vi "LimitSetting.vi"(8 "error in (no error)":errorcluster, 10 "operation":enum16{"Add", "Delete", "Modify"}(ring), 11 "TestSetup in":refnum<class "TestSetup.lvclass">) -> (0 "error out":errorcluster, 3 "TestSetup out":refnum<class "TestSetup.lvclass">)   [LabVIEW 2019, in "TestSetup.lvlib" / "TestSetup.lvclass"]
uses:
  TestSetup.lvclass
  Limit.ctl
  TestSetup.lvclass/TestSetup.ctl
panel:
  in  "OK":bool
  in  "Cancel":bool
  in  "Limit":T1
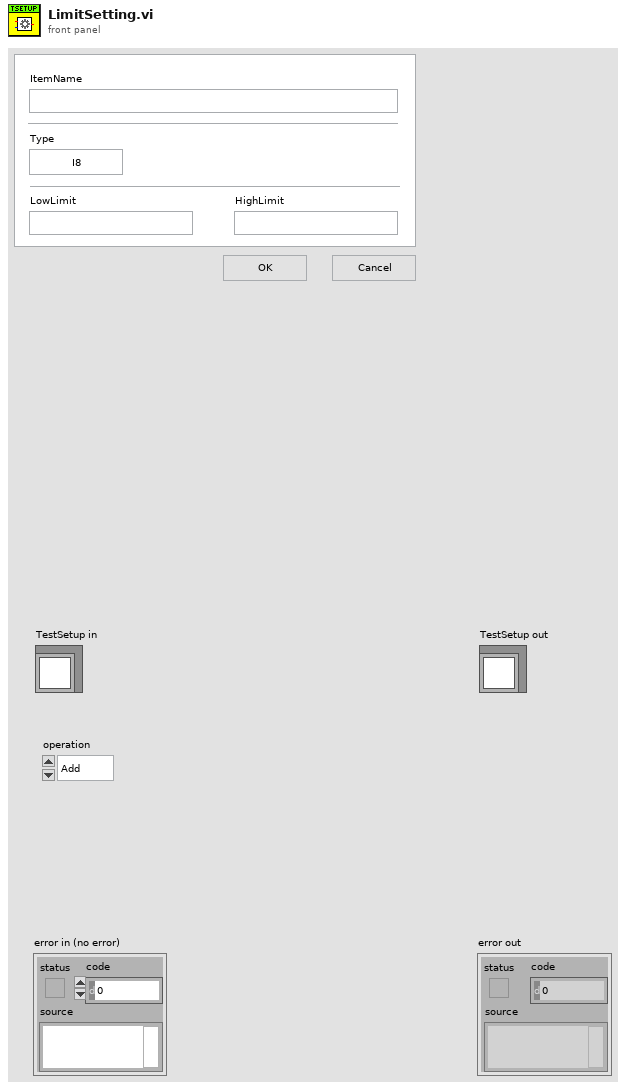
[diagram p1: front panel]
types:
  T1 = typedef "TestSetup.lvlib/TestSetup.lvclass/Limit.ctl" = cluster{"ItemName":string, "Type":enum16{"I8", "I16", "I32", "I64", "U8", "U16", "U32", "U64", "Double Float", "Boolean", "String", "Numeric Array", "String Array"}, "LowLimit":string, "HighLimit":string}
  T2 = enum32{"Invalid", "Standard", "Closed", "Hidden", "Minimized", "Maximized"}
  T3 = enum32{"invalid app kind", "Development System", "Run Time System", "Student Edition", "Embedded LabVIEW", "Evaluation", "Custom"}
  T4 = cluster{"Core":cluster{"Current VI Reference":refnum<vi>, "Close Panel on Exit?":bool}, "Multicolumn Listbox":refnum<vi>, "operation":enum16{"Add", "Delete", "Modify"}, "Limit":refnum<vi>}
  T5 = cluster{"Current VI Reference":refnum<vi>, "Close Panel on Exit?":bool}
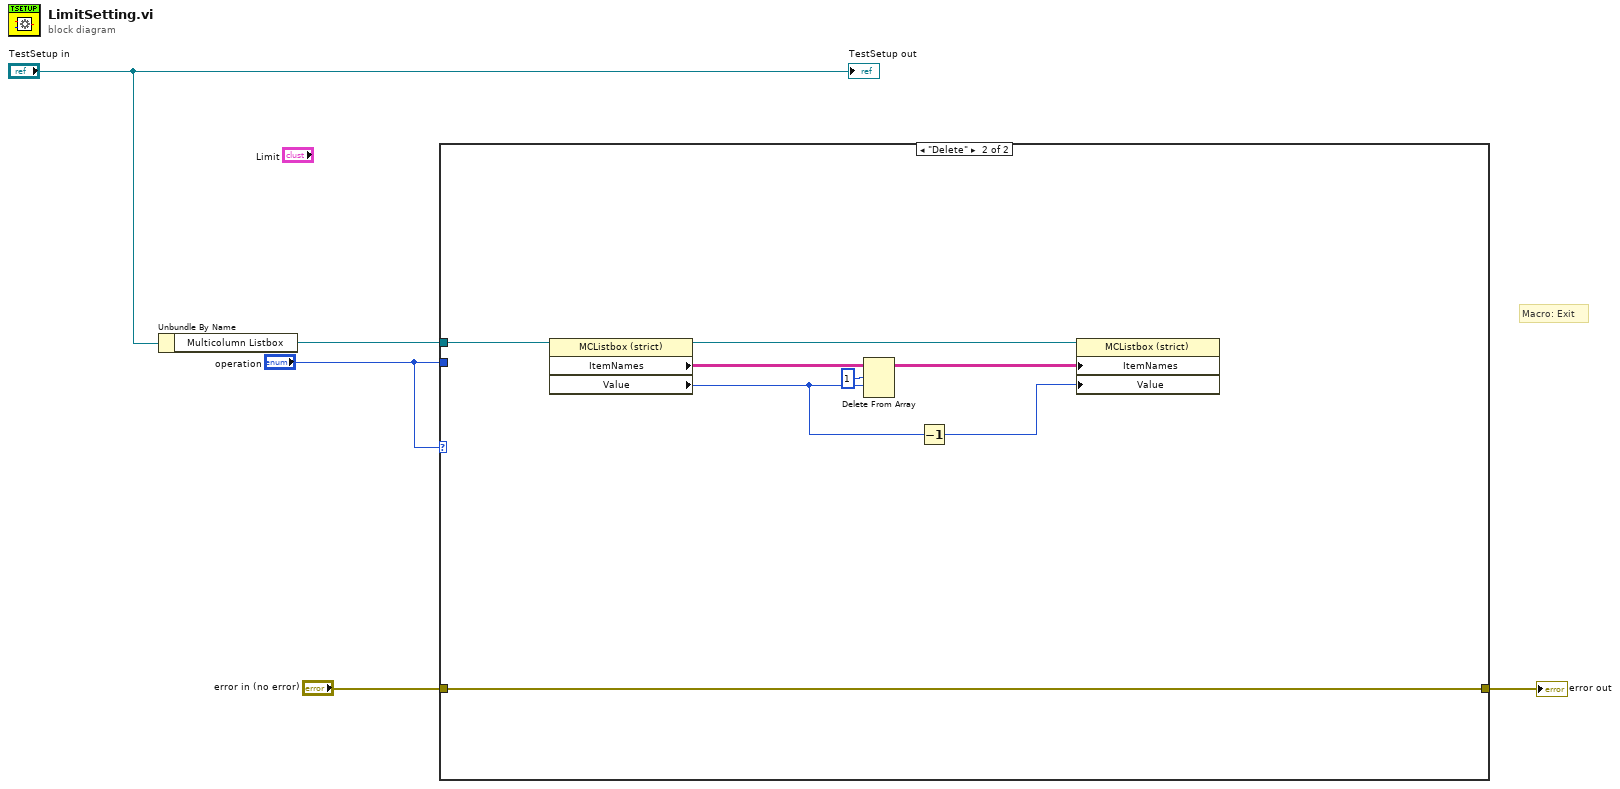
[diagram p0: block diagram]
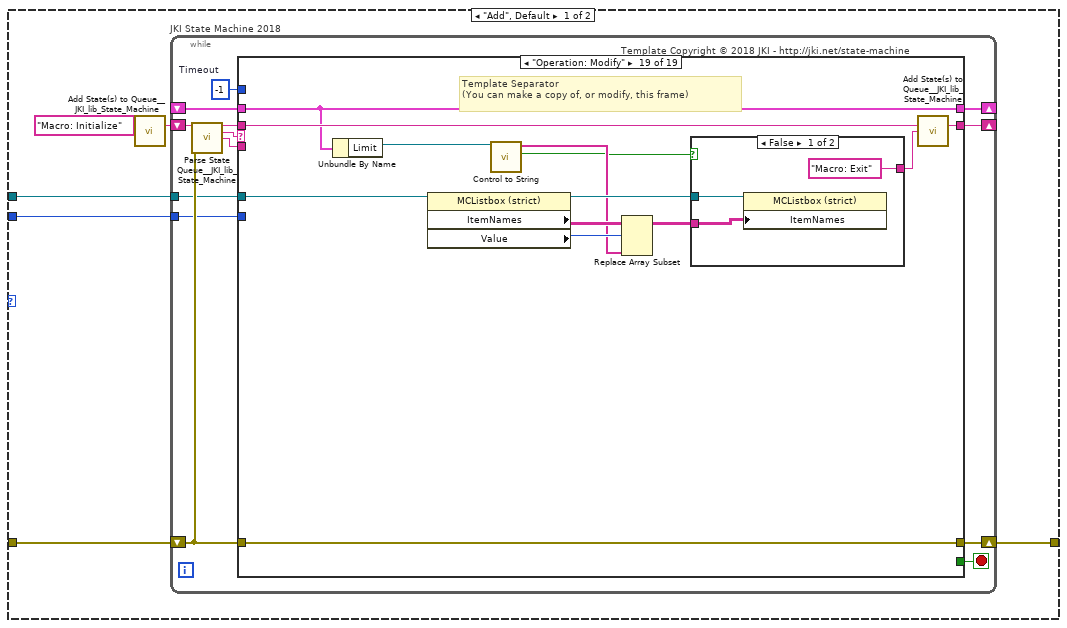
[diagram p2: hidden frame]
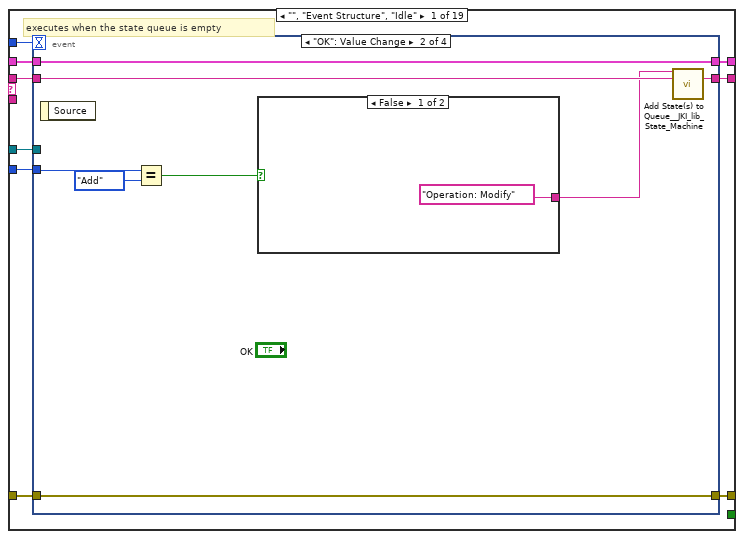
[diagram p3: hidden frame]
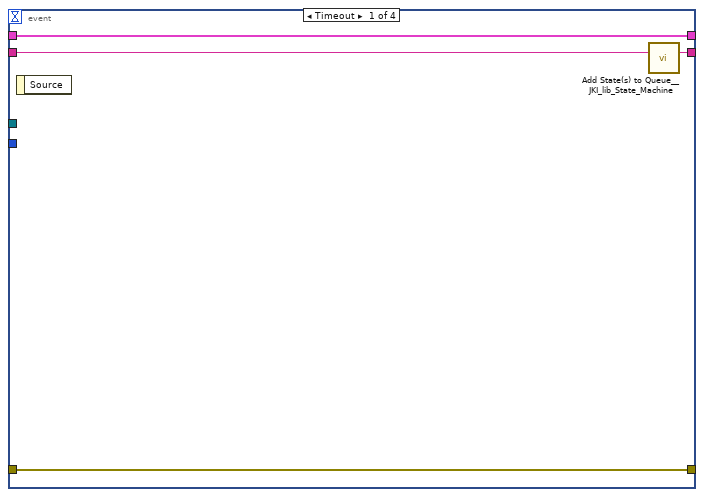
[diagram p4: hidden frame]
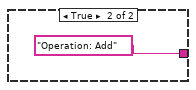
[diagram p5: hidden frame]
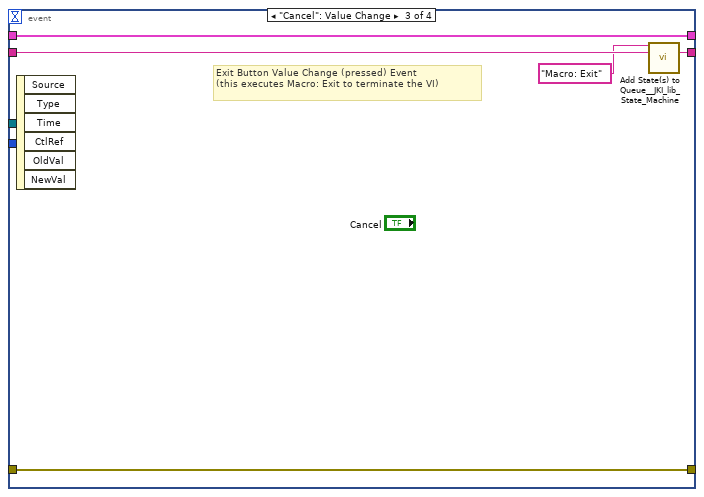
[diagram p6: hidden frame]
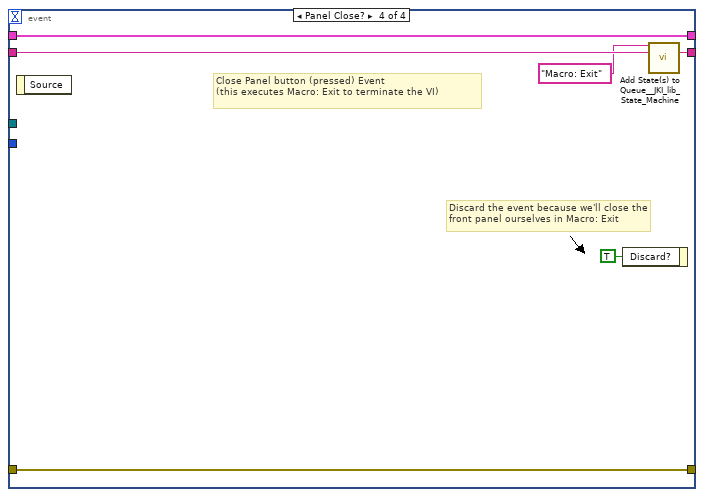
[diagram p7: hidden frame]
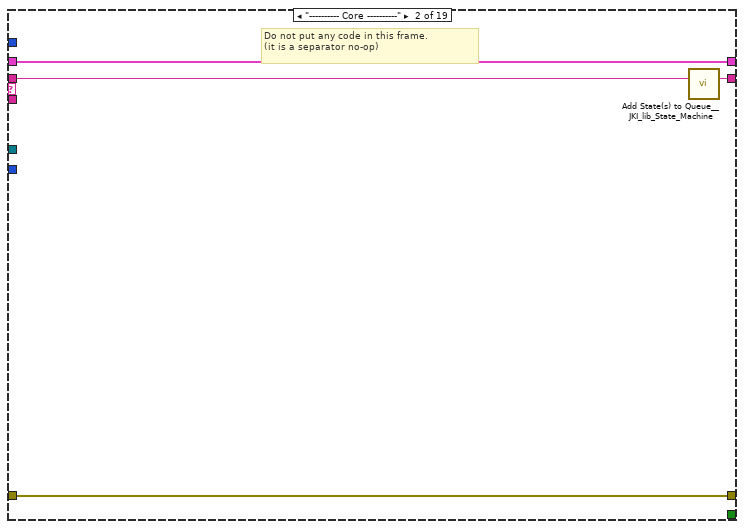
[diagram p8: hidden frame]
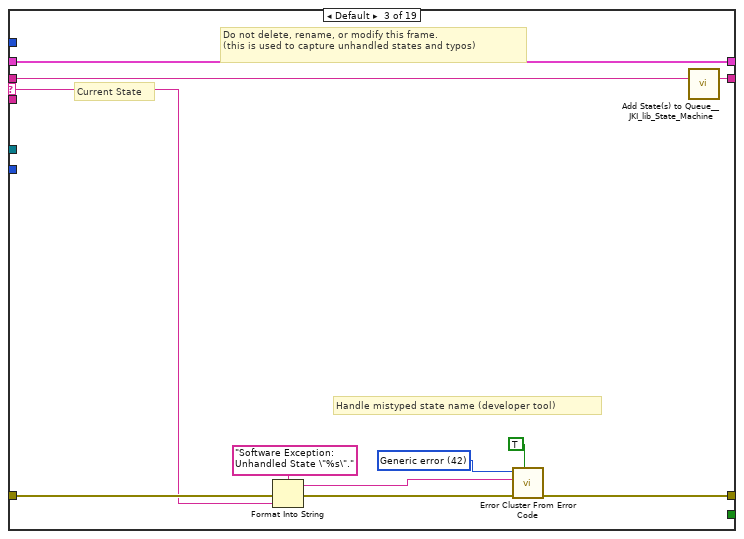
[diagram p9: hidden frame]
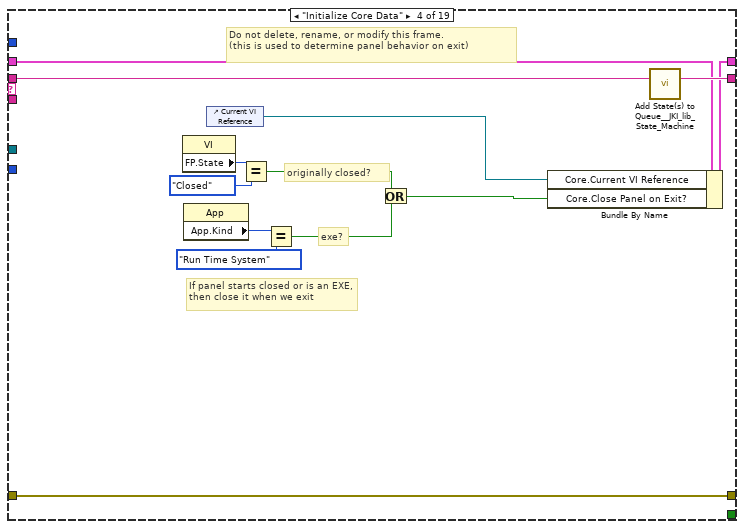
[diagram p10: hidden frame]
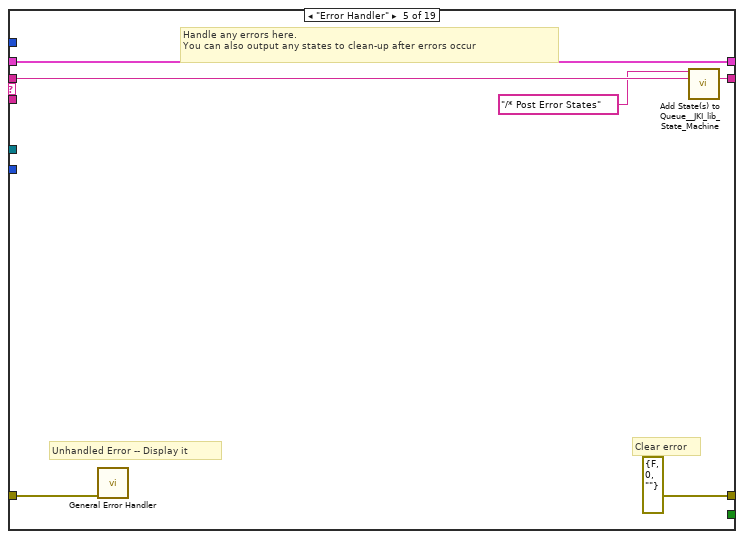
[diagram p11: hidden frame]
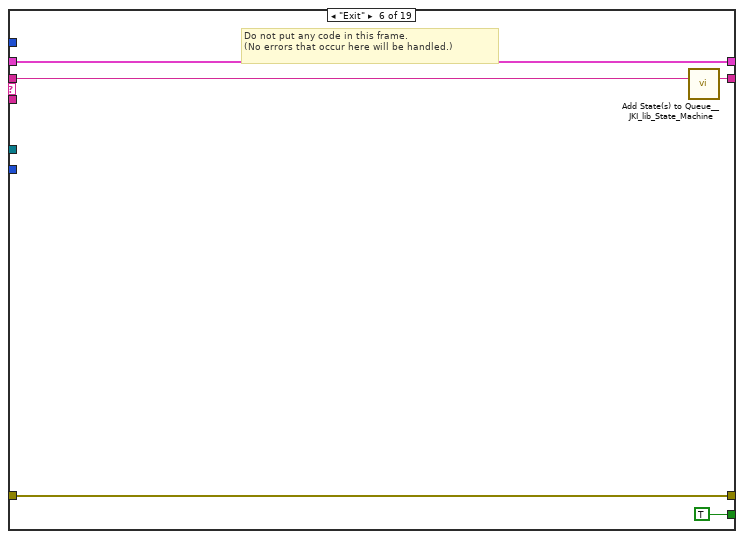
[diagram p12: hidden frame]
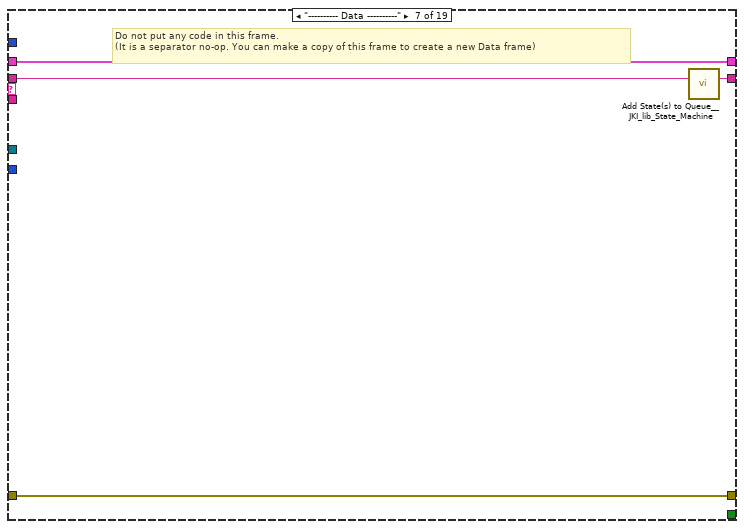
[diagram p13: hidden frame]
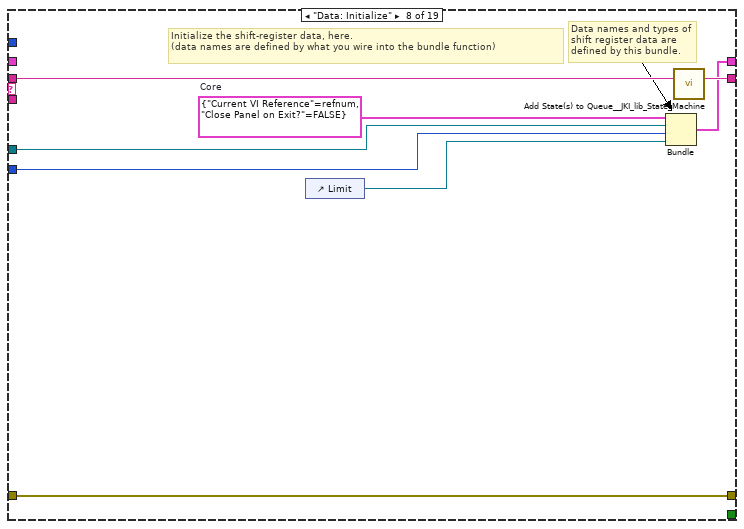
[diagram p14: hidden frame]
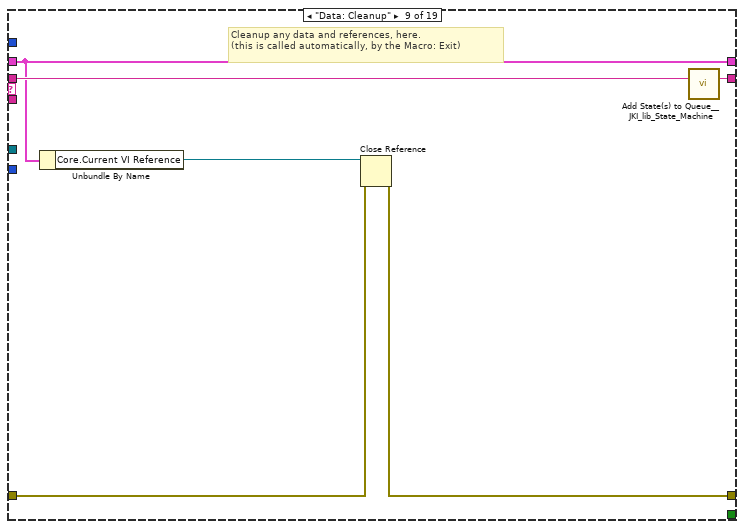
[diagram p15: hidden frame]
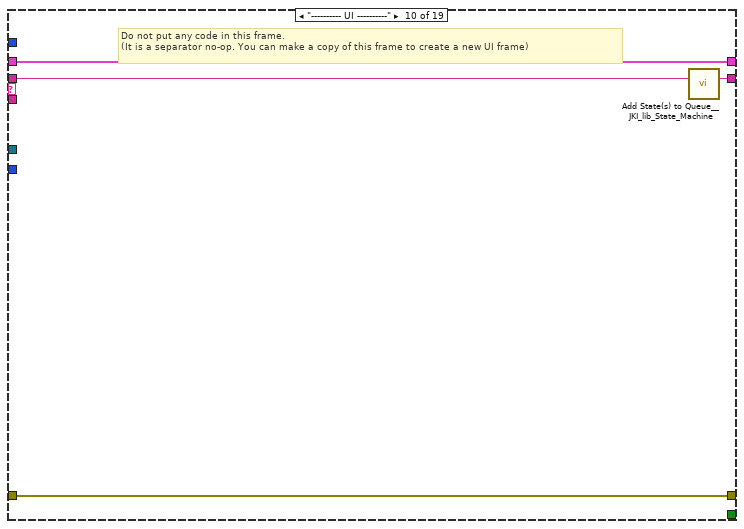
[diagram p16: hidden frame]
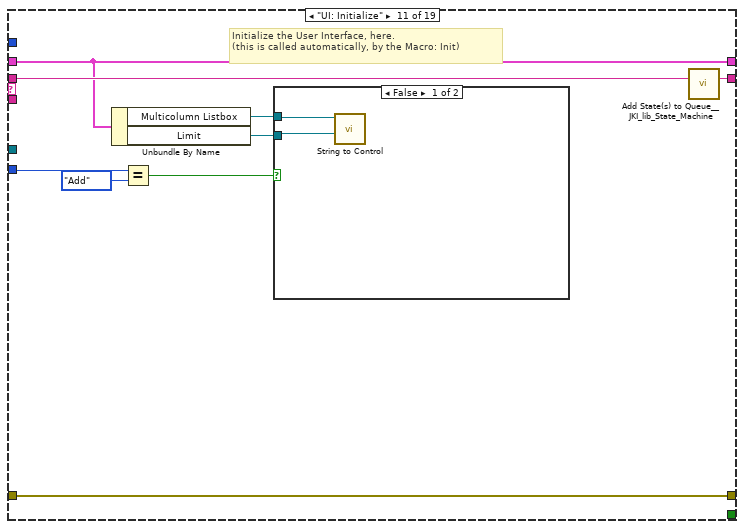
[diagram p17: hidden frame]
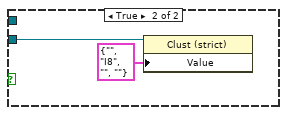
[diagram p18: hidden frame]
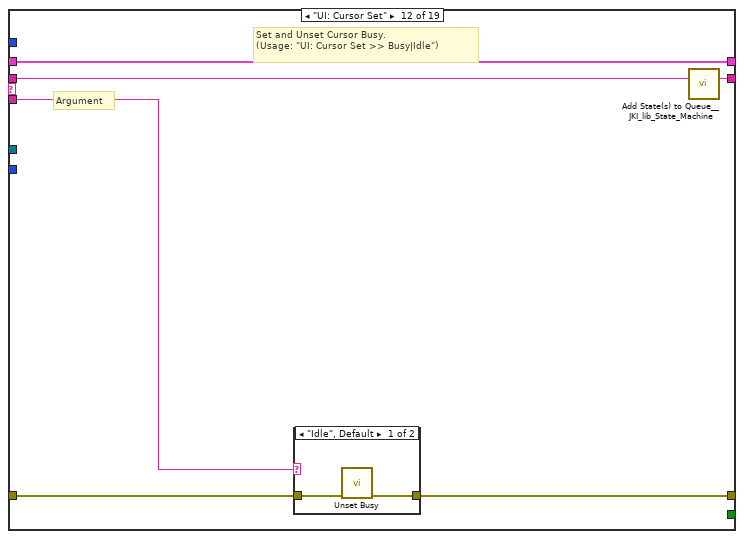
[diagram p19: hidden frame]
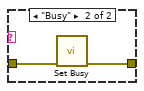
[diagram p20: hidden frame]
diagram:
  # "Macro: Exit"
  n1 = Unbundle By Name("TestSetup in") -> ("Multicolumn Listbox"=w2:refnum<vi>)
  n2 = case shown="\"Delete\"" "operation" {
    tunnel: "error in (no error)" -> [w9 w273]
    tunnel: [w8 w273] -> w3
    tunnel: w2 -> [w7 w276]
    tunnel: "operation" -> [w6 _]
    frame "Add", Default {
      n3 = call <vilib>:"Add State(s) to Queue__JKI_lib_State_Machine.vi"("State(s) in (\"\")"="Macro: Initialize") -> ("States Out"=w11:string)  [unwired: 14 in]
      n4 = while "JKI State Machine 2018" {
        shift-right: [w17] -> _
        shift-left: _ -> [w16]
        shift-right: [w20] -> w8
        shift-left: w9 -> [w14]
        shift-right: [w19] -> _
        shift-left: w11 -> [w21]
        tunnel: w7 -> [w13]
        tunnel: w6 -> [w12]
        stop <- w18 stop-if-true
        w15 = -1  # Timeout
        # "Template Copyright © 2018 JKI - http://jki.net/state-machine"
        n5 = call <vilib>:"Parse State Queue__JKI_lib_State_Machine.vi"("State Queue"=w21, "Error In (no error)"=w14) -> ("Remaining States"=w23:string, "Current State"=w24:string, "Arguments"=w22:string)  [unwired: 11 in]
        n6 = case shown="\"Operation: Modify\"" w24 {
          selector: w24 -> [_ _ w63 _ _ _ _ _ _ _ _ _ _ _ _ _ _ _ _]
          tunnel: w23 -> [w33 w62 w67 w86 w92 w97 w101 w109 w115 w119 w128 w138 w149 w218 w223 w233 w237 w249 w265]
          tunnel: w22 -> [_ _ _ _ _ _ _ _ _ _ _ w133 w143 _ _ _ _ _ _]
          tunnel: w16 -> [w31 w59 w65 w79 w89 w95 w98 _ w110 w116 w125 w136 w145 w215 w220 w230 w234 w246 w258]
          tunnel: [w30 w60 w69 w83 errorcluster {"status"=FALSE, "code"=0, "source"=""} ("error out") w94 w99 w106 w111 w117 w126 w134 w146 w216 w221 w231 w235 w247 w263] -> w20
          tunnel: w14 -> [w29 w60 w68 w83 w88 w94 w99 w106 w112 w117 w126 w135 w147 w216 w221 w231 w235 w247 w263]
          tunnel: [w32 w61 w66 w85 w91 w96 w100 w108 w114 w118 w127 w137 w148 w217 w222 w232 w236 w248 w264] -> w19
          tunnel: [_ _ _ _ _ TRUE _ _ _ _ _ _ _ _ _ _ _ _ _] -> w18
          tunnel: [w28 w59 w65 w84 w89 w95 w98 w107 w110 w116 w125 w136 w145 w215 w220 w230 w234 w246 w258] -> w17
          tunnel: w15 -> [w27 _ _ _ _ _ _ _ _ _ _ _ _ _ _ _ _ _ _]
          tunnel: w13 -> [w26 _ _ _ _ _ _ w104 _ _ _ _ _ _ _ _ _ w244 w257]
          tunnel: w12 -> [w25 _ _ _ _ _ _ w103 _ _ w124 _ _ _ _ _ _ _ _]
          frame "", "Event Structure", "Idle" {
            # "executes when the state queue is empty"
            n7 = event shown="[1] \"OK\": Value Change" {
              selector: _ -> [_ _ _ _]
              dyn-events: _ -> [_ _ _ _]
              timeout: w27 -> [_ _ _ _]
              tunnel: w33 -> [w37 w45 w52 w58]
              tunnel: [w36 w44 w51 w57] -> w32
              tunnel: w31 -> [w34 w42 w49 w55]
              tunnel: [w35 w43 w50 w56] -> w30
              tunnel: w29 -> [w35 w43 w50 w56]
              tunnel: [w34 w42 w49 w55] -> w28
              tunnel: w26 -> [_ _ _ _]
              tunnel: w25 -> [_ w40 _ _]
              event Timeout {
                n8 = event-data() -> ()  [unwired: 1 in, 1 out]
                n9 = call <vilib>:"Add State(s) to Queue__JKI_lib_State_Machine.vi"("State(s) in (\"\")"=w37) -> ("States Out"=w36:string)  [unwired: 14 in]
              }
              event "OK": Value Change {
                n10 = event-data() -> ()  [unwired: 1 in, 1 out]
                n11 = Equal?(x=w40, y=enum16{"Add", "Delete", "Modify"}."Add") -> (x = y?=w38:bool)
                n12 = case shown="False" w38 {
                  tunnel: ["Operation: Modify" "Operation: Add"] -> w41
                  frame False {
                  }
                  frame True {
                  }
                }
                n13 = call <vilib>:"Add State(s) to Queue__JKI_lib_State_Machine.vi"("State(s) in Front (\"\")"=w41, "State(s) in (\"\")"=w45) -> ("States Out"=w44:string)  [unwired: 13 in]
              }
              event "Cancel": Value Change {
                # "Exit Button Value Change (pressed) Event\n(this executes Macro: Exit to terminate the VI)"
                n14 = event-data() -> ()  [unwired: 1 in, 6 out]
                n15 = call <vilib>:"Add State(s) to Queue__JKI_lib_State_Machine.vi"("State(s) in Front (\"\")"="Macro: Exit", "State(s) in (\"\")"=w52) -> ("States Out"=w51:string)  [unwired: 13 in]
              }
              event Panel Close? {
                # "Discard the event because we'll close the front panel ourselves in Macro: Exit"
                # "Close Panel button (pressed) Event\n(this executes Macro: Exit to terminate the VI)"
                n16 = event-data() -> ()  [unwired: 1 in, 1 out]
                n17 = event-data("Discard?"=TRUE) -> ()  [unwired: 1 in, 1 out]
                n18 = call <vilib>:"Add State(s) to Queue__JKI_lib_State_Machine.vi"("State(s) in Front (\"\")"="Macro: Exit", "State(s) in (\"\")"=w58) -> ("States Out"=w57:string)  [unwired: 13 in]
              }
            }
          }
          frame "---------- Core ----------" {
            # "Do not put any code in this frame.\n(it is a separator no-op)"
            n19 = call <vilib>:"Add State(s) to Queue__JKI_lib_State_Machine.vi"("State(s) in (\"\")"=w62) -> ("States Out"=w61:string)  [unwired: 14 in]
          }
          frame Default {
            w72 = 42 items=["No error", "Argument error", "Memory is full", "Out of zone", "End of file", "File already open", "Generic file I/O error", "File not found", "File permission error", "Disk is full", "Duplicate path", "Too many files open", "System feature not enabled", "Resource file not found", "Cannot add resource", "Resource not found", "Image not found", "Image memory error", "Pen does not exist", "Config type invalid", "Config token not found", "Config parse error", "Config memory error", "Bad external code format", "Bad external code offset", "External code not present", "Null window", "Destroy window error", "Null menu", "Print aborted", "Bad print record", "Print driver error", "Windows error during printing", "Memory error during printing", "Print dialog error", "Generic print error", "Invalid device refnum", "Device not found", "Device parameter error", "Device unit error", "Cannot open device", "Device call aborted", "Generic error", "Cancelled by user", "Object ID too low", "Object ID too high", "Object not in heap", "Unknown heap", "Unknown object (invalid DefProc)", "Unknown object (DefProc not in table)", "Message out of range", "Invalid (null) method", "Unknown message", "Manager call not supported", "Bad address", "Network operation in progress", "Network operation timed out", "Connection is busy", "Network attribute not supported", "Network error", "Address in use", "System out of memory", "Connection aborted", "Connection refused", "Not connected", "Already connected", "Connection closed", "Initialization error (interapplication manager)", "Bad occurrence", "Wait on unbound occurrence handler", "Occurrence queue overflow", "Datalog type conflict", "Unused", "Unrecognized type (interapplication manager)", "Memory corrupt", "Failed to make temporary DLL", "Old CIN version", "Drag socket not found", "Failed to load drop-object", "Failed to register OLE object", "Failed to release OLE object", "Format specifier type mismatch", "Unknown format specifier", "Too few format specifiers", "Too many format specifiers", "Scan failed", "Newer CIN version", "Error converting to variant", "Runtime menu error", "Password tampered", "Variant attribute not found", "Incompatible variant data type", "Event data is not available", "Event Store is not present", "Occurrence is not found", "Event Queue is not created", "Event info is not available", "Refnum passed is NULL", "Error retrieving Class GUID", "Error retrieving CoClass GUID", "Error retrieving TypeLib GUID.", "Bad built application magic bytes.", "Specific driver is different from the specific driver associated with the Logical Name.", "There is no session opened to the class driver.", "Max Error", "MAX - Error with config objects", "MAX - Error loading configuration", "MAX - Group not supported"]
            # "Current State"
            # "Do not delete, rename, or modify this frame.\n(this is used to capture unhandled states and typos)"
            # "Handle mistyped state name (developer tool)"
            n20 = Format Into String(format string="Software Exception: Unhandled State \"%s\"." ("message"), error in=w68, w63) -> (resulting string=w71:string, error out=w70:errorcluster)  [unwired: 1 in]
            n21 = call <vilib>:"Error Cluster From Error Code.vi"("show call chain? (False)"=TRUE, "error in (no error)"=w70, "error message (\"\")"=w71, "error code (0)"=w72) -> ("error out"=w69:errorcluster)  [unwired: 5 in]
            n22 = call <vilib>:"Add State(s) to Queue__JKI_lib_State_Machine.vi"("State(s) in (\"\")"=w67) -> ("States Out"=w66:string)  [unwired: 14 in]
          }
          frame "Initialize Core Data" {
            # "Do not delete, rename, or modify this frame.\n(this is used to determine panel behavior on exit)"
            # "originally closed?"
            # "exe?"
            # "If panel starts closed or is an EXE, then close it when we exit"
            n23 = property class="VI"() -> ("FP.State"=w76:T2)  [unwired: 2 in, 2 out]
            n24 = property class="App"() -> ("App.Kind"=w82:T3)  [unwired: 2 in, 2 out]
            n25 = control-ref of="Current VI Reference"() -> (w77:refnum<vi>)
            n26 = Equal?(x=w76, y=T2."Closed" ("Front Panel Window:State")) -> (x = y?=w74:bool)
            n27 = Equal?(x=w82, y=T3."Run Time System" ("Application:Kind")) -> (x = y?=w80:bool)
            n28 = Or(x=w74, y=w80) -> (x .or. y?=w78:bool)
            n29 = Bundle By Name(cluster=w79, "Core.Current VI Reference"=w77, "Core.Close Panel on Exit?"=w78) -> (w84:T4)
            n30 = call <vilib>:"Add State(s) to Queue__JKI_lib_State_Machine.vi"("State(s) in (\"\")"=w86) -> ("States Out"=w85:string)  [unwired: 14 in]
          }
          frame "Error Handler" {
            # "Unhandled Error -- Display it"
            # "Handle any errors here.\nYou can also output any states to clean-up after errors occur"
            # "Clear error"
            n31 = call <vilib>:"General Error Handler.vi"("error in (no error)"=w88) -> ()  [unwired: 10 in, 5 out]
            n32 = call <vilib>:"Add State(s) to Queue__JKI_lib_State_Machine.vi"("State(s) in Front (\"\")"="/* Post Error States", "State(s) in (\"\")"=w92) -> ("States Out"=w91:string)  [unwired: 13 in]
          }
          frame "Exit" {
            # "Do not put any code in this frame.\n(No errors that occur here will be handled.)"
            n33 = call <vilib>:"Add State(s) to Queue__JKI_lib_State_Machine.vi"("State(s) in (\"\")"=w97) -> ("States Out"=w96:string)  [unwired: 14 in]
          }
          frame "---------- Data ----------" {
            # "Do not put any code in this frame.\n(It is a separator no-op. You can make a copy of this frame to create a new Data frame)"
            n34 = call <vilib>:"Add State(s) to Queue__JKI_lib_State_Machine.vi"("State(s) in (\"\")"=w101) -> ("States Out"=w100:string)  [unwired: 14 in]
          }
          frame "Data: Initialize" {
            w105 = T5 {"Current VI Reference"=refnum, "Close Panel on Exit?"=FALSE}  # Core
            # "Data names and types of shift register data are defined by this bundle."
            # "Initialize the shift-register data, here.\n(data names are defined by what you wire into the bundle function)"
            n35 = control-ref of="Limit"() -> (w102:refnum<vi>)
            n36 = Bundle("Core"=w105, "Multicolumn Listbox"=w104, "operation"=w103, "Limit"=w102) -> (w107:T4)  [unwired: 1 in]
            n37 = call <vilib>:"Add State(s) to Queue__JKI_lib_State_Machine.vi"("State(s) in (\"\")"=w109) -> ("States Out"=w108:string)  [unwired: 14 in]
          }
          frame "Data: Cleanup" {
            # "Cleanup any data and references, here.\n(this is called automatically, by the Macro: Exit)"
            n38 = Unbundle By Name(w110) -> ("Core.Current VI Reference"=w113:refnum<vi>)
            n39 = Close Reference(reference=w113, error in (no error)=w112) -> (error out=w111:errorcluster)
            n40 = call <vilib>:"Add State(s) to Queue__JKI_lib_State_Machine.vi"("State(s) in (\"\")"=w115) -> ("States Out"=w114:string)  [unwired: 14 in]
          }
          frame "---------- UI ----------" {
            # "Do not put any code in this frame.\n(It is a separator no-op. You can make a copy of this frame to create a new UI frame)"
            n41 = call <vilib>:"Add State(s) to Queue__JKI_lib_State_Machine.vi"("State(s) in (\"\")"=w119) -> ("States Out"=w118:string)  [unwired: 14 in]
          }
          frame "UI: Initialize" {
            # "Initialize the User Interface, here.\n(this is called automatically, by the Macro: Init)"
            n42 = Unbundle By Name(w125) -> ("Multicolumn Listbox"=w120:refnum<vi>, "Limit"=w122:refnum<vi>)
            n43 = Equal?(x=w124, y=enum16{"Add", "Delete", "Modify"}."Add") -> (x = y?=w121:bool)
            n44 = case shown="False" w121 {
              tunnel: w122 -> [w129 w132]
              tunnel: w120 -> [w130 _]
              frame False {
                n45 = call "String to Control.vi"("Limit"=w129, "Multicolumn Listbox"=w130) -> ()  [unwired: 10 in]
              }
              frame True {
                n46 = property class="Clust (strict)"(reference=w132, "Value"=T1 {"ItemName"="", "Type"=enum."I8", "LowLimit"="", "HighLimit"=""}) -> ()  [unwired: 1 in, 2 out]
              }
            }
            n47 = call <vilib>:"Add State(s) to Queue__JKI_lib_State_Machine.vi"("State(s) in (\"\")"=w128) -> ("States Out"=w127:string)  [unwired: 14 in]
          }
          frame "UI: Cursor Set" {
            # "Argument"
            # "Set and Unset Cursor Busy.\n(Usage: \"UI: Cursor Set >> Busy|Idle\")"
            n48 = case shown="\"Idle\", Default" w133 {
              tunnel: w135 -> [w140 w142]
              tunnel: [w139 w141] -> w134
              frame "Idle", Default {
                n49 = call <vilib>:"Unset Busy.vi"("error in (no error)"=w140) -> ("error out"=w139:errorcluster)  [unwired: 10 in]
              }
              frame "Busy" {
                n50 = call <vilib>:"Set Busy.vi"("error in (no error)"=w142) -> ("error out"=w141:errorcluster)  [unwired: 9 in, 1 out]
              }
            }
            n51 = call <vilib>:"Add State(s) to Queue__JKI_lib_State_Machine.vi"("State(s) in (\"\")"=w138) -> ("States Out"=w137:string)  [unwired: 14 in]
          }
          frame "UI: Front Panel State" {
            # "Argument"
            # "Set Front Panel Open or Closed\n(Usage: \"UI: Front Panel State >> Open|Close\")"
            n52 = Unbundle By Name(w145) -> ("Core.Current VI Reference"=w144:refnum<vi>)
            n53 = case shown="\"Minimize\", \"Minimized\"" w143 {
              tunnel: w147 -> [w155 w170 w181 w194 w207]
              tunnel: [w157 w171 w183 w196 w209] -> w146
              tunnel: w144 -> [w156 w168 w182 w195 w208]
              frame "Open", "Standard", Default {
                w150 = T2."Standard" ("State")
                n54 = property class="VI"(reference=w156, error in=w155) -> (reference out=w153:refnum<vi>, error out=w154:errorcluster, "FP.State"=w152:T2)
                n55 = Not Equal?(x=w152, y=w150) -> (x != y?=w151:bool)
                n56 = case shown="True" w151 {
                  tunnel: [w161 w163] -> w157
                  tunnel: w154 -> [w160 w163]
                  tunnel: w153 -> [w159 _]
                  tunnel: w150 -> [w158 _]
                  frame True {
                    n57 = invoke class="VI" method="FP.Open"(reference=w159, error in=w160, "Activate"=TRUE, "State"=w158) -> (error out=w161:errorcluster)  [unwired: 1 in, 4 out]
                  }
                  frame False {
                  }
                }
              }
              frame "Close", "Closed" {
                n58 = property class="VI"(reference=w168, error in=w170) -> (reference out=w167:refnum<vi>, error out=w169:errorcluster, "FP.State"=w165:T2)
                n59 = Not Equal?(x=w165, y=T2."Closed" ("Front Panel Window:State")) -> (x != y?=w164:bool)
                n60 = case shown="True" w164 {
                  tunnel: [w172 w175] -> w171
                  tunnel: w169 -> [w172 w174]
                  tunnel: w167 -> [_ w173]
                  frame False {
                  }
                  frame True {
                    n61 = invoke class="VI" method="FP.Close"(reference=w173, error in=w174) -> (error out=w175:errorcluster)  [unwired: 1 in, 2 out]
                  }
                }
              }
              frame "Hidden", "Hide" {
                w176 = T2."Hidden" ("State")
                n62 = property class="VI"(reference=w182, error in=w181) -> (reference out=w179:refnum<vi>, error out=w180:errorcluster, "FP.State"=w178:T2)
                n63 = Not Equal?(x=w178, y=w176) -> (x != y?=w177:bool)
                n64 = case shown="True" w177 {
                  tunnel: [w187 w188] -> w183
                  tunnel: w180 -> [w186 w188]
                  tunnel: w179 -> [w185 _]
                  tunnel: w176 -> [w184 _]
                  frame True {
                    n65 = invoke class="VI" method="FP.Open"(reference=w185, error in=w186, "State"=w184) -> (error out=w187:errorcluster)  [unwired: 2 in, 4 out]
                  }
                  frame False {
                  }
                }
              }
              frame "Minimize", "Minimized" {
                w189 = T2."Minimized" ("State")
                n66 = property class="VI"(reference=w195, error in=w194) -> (reference out=w192:refnum<vi>, error out=w193:errorcluster, "FP.State"=w191:T2)
                n67 = Not Equal?(x=w191, y=w189) -> (x != y?=w190:bool)
                n68 = case shown="True" w190 {
                  tunnel: [w200 w201] -> w196
                  tunnel: w193 -> [w199 w201]
                  tunnel: w192 -> [w198 _]
                  tunnel: w189 -> [w197 _]
                  frame True {
                    n69 = invoke class="VI" method="FP.Open"(reference=w198, error in=w199, "State"=w197) -> (error out=w200:errorcluster)  [unwired: 2 in, 4 out]
                  }
                  frame False {
                  }
                }
              }
              frame "Maximize", "Maximized" {
                w202 = T2."Maximized" ("State")
                n70 = property class="VI"(reference=w208, error in=w207) -> (reference out=w205:refnum<vi>, error out=w206:errorcluster, "FP.State"=w204:T2)
                n71 = Not Equal?(x=w204, y=w202) -> (x != y?=w203:bool)
                n72 = case shown="True" w203 {
                  tunnel: [w213 w214] -> w209
                  tunnel: w206 -> [w212 w214]
                  tunnel: w205 -> [w211 _]
                  tunnel: w202 -> [w210 _]
                  frame True {
                    n73 = invoke class="VI" method="FP.Open"(reference=w211, error in=w212, "State"=w210) -> (error out=w213:errorcluster)  [unwired: 2 in, 4 out]
                  }
                  frame False {
                  }
                }
              }
            }
            n74 = call <vilib>:"Add State(s) to Queue__JKI_lib_State_Machine.vi"("State(s) in (\"\")"=w149) -> ("States Out"=w148:string)  [unwired: 14 in]
          }
          frame "---------- Macro ----------" {
            # "Do not put any code in this frame.\n(It is a separator no-op. You can make a copy of this frame to create a new Macro frame)"
            n75 = call <vilib>:"Add State(s) to Queue__JKI_lib_State_Machine.vi"("State(s) in (\"\")"=w218) -> ("States Out"=w217:string)  [unwired: 14 in]
          }
          frame "Macro: Initialize" {
            w219 = "Data: Initialize\nInitialize Core Data\nUI: Initialize\nUI: Front Panel State >> Open"  # Data: Initialize Initialize Core Data UI: Initialize UI: Front Panel State >> Open
            # "Initialization Macro\n(This is called once, when the VI starts)"
            n76 = call <vilib>:"Add State(s) to Queue__JKI_lib_State_Machine.vi"("State(s) in Front (\"\")"=w219, "State(s) in (\"\")"=w223) -> ("States Out"=w222:string)  [unwired: 13 in]
          }
          frame "Macro: Exit" {
            # "Exit Macro\n(This is called once, when the VI exits)"
            n77 = Unbundle By Name(w230) -> ("Core.Close Panel on Exit?"=w229:bool)
            n78 = Select(t="UI: Front Panel State >> Close", s=w229, f="") -> (s? t:f=w226:string)
            n79 = call <vilib>:"Add State(s) to Queue__JKI_lib_State_Machine.vi"("State(s) in (\"\")"=w226, "State(s) at Back (\"\")"="Data: Cleanup\nExit") -> ("States Out"=w224:string)  [unwired: 13 in]
            n80 = call <vilib>:"Add State(s) to Queue__JKI_lib_State_Machine.vi"("State(s) in Front (\"\")"=w224, "State(s) in (\"\")"=w233) -> ("States Out"=w232:string)  [unwired: 13 in]
          }
          frame "---------- Operation ----------" {
            # "Template Separator\n(You can make a copy of, or modify, this frame)"
            n81 = call <vilib>:"Add State(s) to Queue__JKI_lib_State_Machine.vi"("State(s) in (\"\")"=w237) -> ("States Out"=w236:string)  [unwired: 14 in]
          }
          frame "Operation: Add" {
            # "Template Separator\n(You can make a copy of, or modify, this frame)"
            n82 = Unbundle By Name(w246) -> ("Limit"=w245:refnum<vi>)
            n83 = property class="MCListbox (strict)"(reference=w244) -> (reference out=w243:refnum<vi>, "ItemNames"=w242:string[][])  [unwired: 1 in, 1 out]
            n84 = call "Control to String.vi"("Limit"=w245) -> ("error"=w239:bool, "StringLimit"=w240:string[])  [unwired: 8 in, 1 out]
            n85 = Build Array (concatenate)(w242, w240) -> (w241:string[][])
            n86 = case shown="False" w239 {
              tunnel: w243 -> [w252 _]
              tunnel: w241 -> [w251 _]
              tunnel: ["Macro: Exit" _] -> w238
              frame False {
                n87 = property class="MCListbox (strict)"(reference=w252, "ItemNames"=w251) -> ()  [unwired: 1 in, 2 out]
              }
              frame True {
              }
            }
            n88 = call <vilib>:"Add State(s) to Queue__JKI_lib_State_Machine.vi"("State(s) in (\"\")"=w249, "State(s) at Back (\"\")"=w238) -> ("States Out"=w248:string)  [unwired: 13 in]
          }
          frame "Operation: Modify" {
            # "Template Separator\n(You can make a copy of, or modify, this frame)"
            n89 = Unbundle By Name(w258) -> ("Limit"=w262:refnum<vi>)
            n90 = property class="MCListbox (strict)"(reference=w257) -> (reference out=w261:refnum<vi>, "ItemNames"=w260:string[][], "Value"=w256:i32)  [unwired: 1 in, 1 out]
            n91 = call "Control to String.vi"("Limit"=w262) -> ("error"=w254:bool, "StringLimit"=w255:string[])  [unwired: 8 in, 1 out]
            n92 = Replace Array Subset(array=w260, new element=w255, index (row)=w256) -> (w259:string[][])  [unwired: 1 in]
            n93 = case shown="False" w254 {
              tunnel: w261 -> [w268 _]
              tunnel: w259 -> [w267 _]
              tunnel: ["Macro: Exit" _] -> w253
              frame False {
                n94 = property class="MCListbox (strict)"(reference=w268, "ItemNames"=w267) -> ()  [unwired: 1 in, 2 out]
              }
              frame True {
              }
            }
            n95 = call <vilib>:"Add State(s) to Queue__JKI_lib_State_Machine.vi"("State(s) in (\"\")"=w265, "State(s) at Back (\"\")"=w253) -> ("States Out"=w264:string)  [unwired: 13 in]
          }
        }
      }
    }
    frame "Delete" {
      n96 = property class="MCListbox (strict)"(reference=w276) -> (reference out=w272:refnum<vi>, "ItemNames"=w275:string[][], "Value"=w270:i32)  [unwired: 1 in, 1 out]
      n97 = Delete From Array(array=w275, length=1, index (row)=w270) -> (array with subset deleted=w271:string[][])  [unwired: 1 in, 1 out]
      n98 = Decrement(x=w270) -> (x-1=w269:i32)
      n99 = property class="MCListbox (strict)"(reference=w272, "ItemNames"=w271, "Value"=w269) -> ()  [unwired: 1 in, 2 out]
    }
  }
  "error out" <- w3
  "TestSetup out" <- "TestSetup in"
